vi "MagReadGainSet.vi"(8 "Error in":errorcluster, 10 "Gain Set":enum16{"8.1G", "1.9G"}(ring), 11 "Serial port":refnum<visa-resource-name>="COM13") -> (0 "Error out":errorcluster, 1 "Mag State":bool[](array[boolean]), 2 "B(G)":dbl[][](array[numeric]), 3 "Serial port out":refnum<visa-resource-name>, 4 "Gain Read":enum16{"8.1G", "1.9G"}(ring))   [LabVIEW 2012]
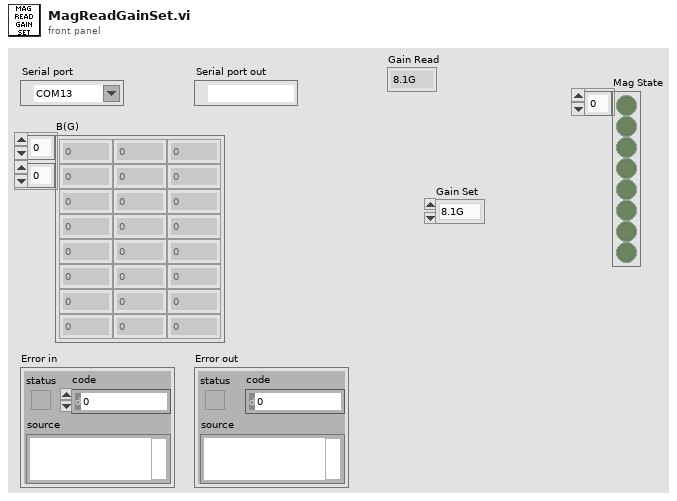
[diagram p1: front panel]
types:
  T1 = enum16{"big-endian, network order", "native, host order", "little-endian"}
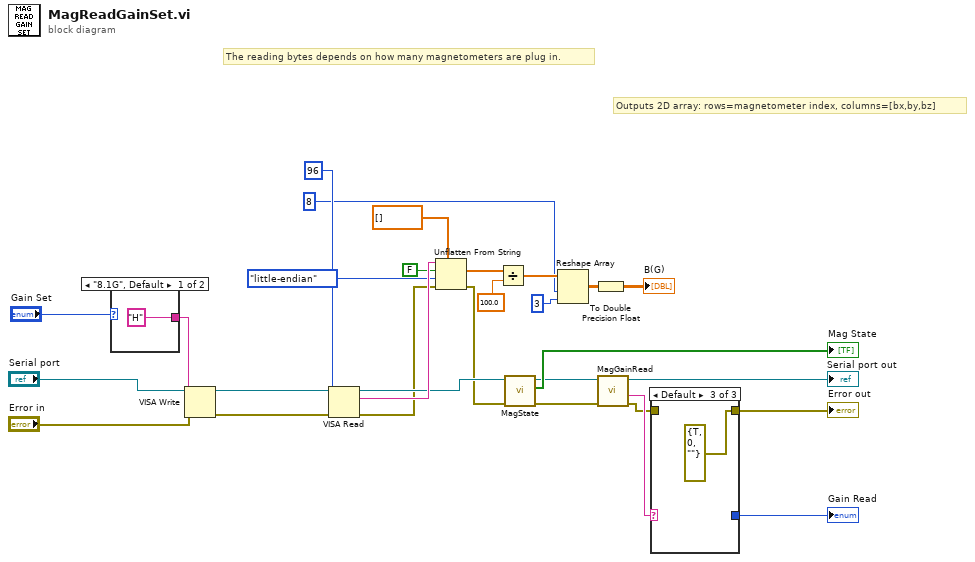
[diagram p0: block diagram]
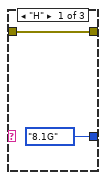
[diagram p2: hidden frame]
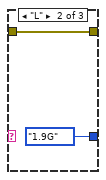
[diagram p3: hidden frame]
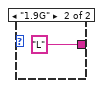
[diagram p4: hidden frame]
diagram:
  # "Outputs 2D array: rows=magnetometer index, columns=[bx,by,bz]"
  # "The reading bytes depends on how many magnetometers are plug in."
  n1 = case shown="\"8.1G\", Default" "Gain Set" {
    tunnel: ["H" ("write buffer") "L" ("write buffer")] -> w10
    frame "8.1G", Default {
    }
    frame "1.9G" {
    }
  }
  n2 = VISA Write(VISA resource name="Serial port", write buffer=w10, error in (no error)="Error in") -> (VISA resource name out=w9:refnum<visa-resource-name>, error out=w8:errorcluster)  [unwired: 1 out]
  n3 = VISA Read(VISA resource name=w9, byte count=u32 96, error in (no error)=w8) -> (VISA resource name out=w15:refnum<visa-resource-name>, read buffer=w29:string, error out=w13:errorcluster)  [unwired: 1 out]
  n4 = Unflatten From String(type=sgl[] [], binary string=w29, data includes array or string size? (T)=FALSE, byte order (0:big-endian, network order)=T1."little-endian", error in (no error)=w13) -> (value=w26:sgl[], error out=w12:errorcluster)  [unwired: 1 out]
  n5 = Divide(x=w26, y=sgl 100.0) -> (x/y=w20:sgl[])
  n6 = call "MagState.vi"("Error in"=w12, "Serial port"=w15) -> ("Error out"=w5:errorcluster, "Mag State"=→"Mag State":bool[], "Serial port out"=w7:refnum<visa-resource-name>)  [unwired: 7 in]
  n7 = Reshape Array(w20, 8 ("byte count"), 3 ("dimension size")) -> (w17:sgl[][])
  n8 = To Double Precision Float(number=w17) -> (double precision float=→"B(G)":dbl[][])
  n9 = call "MagGainRead.vi"("Error in"=w5, "Serial port"=w7) -> ("Error out"=w2:errorcluster, "Gain Read"=w4:string, "Serial port out"=→"Serial port out":refnum<visa-resource-name>)  [unwired: 7 in]
  n10 = case shown="Default" w4 {
    tunnel: [enum16{"8.1G", "1.9G"}."8.1G" ("Gain Read") enum16{"8.1G", "1.9G"}."1.9G" ("Gain Read") _] -> w3
    tunnel: w2 -> [w32 w34 _]
    tunnel: [w32 w34 errorcluster {"status"=TRUE, "code"=0, "source"=""} ("Error out")] -> w1
    frame "H" {
    }
    frame "L" {
    }
    frame Default {
    }
  }
  "Error out" <- w1
  "Gain Read" <- w3
